vi "Controller Top Level.vi"(8 "error in (no error)":errorcluster) -> (0 "error out":errorcluster)   [LabVIEW 2020, in "Controller.lvlib"]
uses:
  Controller.lvlib
  Private Controls/Module Action.ctl
  Public Controls/Module Data Cluster.ctl
  Public Controls/Config.ctl
  c2d6bbf9-d574-4896-9299-2729cd30e33b.vi
  27c827a8-6ce2-46ff-b742-8397f53ceddc.vi
  e3555320-3669-4681-98ae-afe808cba037.vi
  16cb41ff-8f3c-4f22-bc48-50ffacbfc1d7.vi
  <vilib>/Utility/error.llb/Clear Errors.vi
  UI/UI.lvlib
  Error Handler/Error Handler.lvlib
panel:
  out "Action":T1
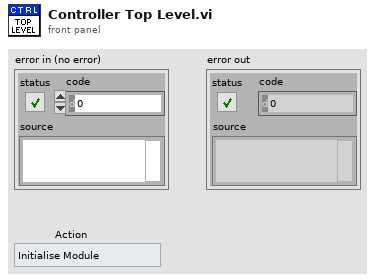
[diagram p1: front panel]
types:
  T1 = typedef "Controller.lvlib/Module Action.ctl" = enum16{"Initialise Module", "Connect", "Setup", "Pause", "Start", "Search Network", "Get Local", "Stop", "Wait: Time Elapsed", "Error", "Exit"}
  T2 = typedef "Controller.lvlib/Module Data Cluster.ctl" = cluster{"Pause?":bool, "Iteration":i32, "Time Elapsed?":bool, "Config":T3, "Local IP":string}
  T3 = typedef "Controller.lvlib/Config.ctl" = cluster{"Value":dbl}
  T4 = typedef "UI.lvlib/IP Address Response Type Def.ctl" = cluster{"Address":string, "Response":string, "Boolean":bool}
  T5 = typedef "UI.lvlib/IP Stats.ctl" = cluster{"Address":string, "Average Response Time":i32, "Loss %":i32, "Min Response Time":i32, "Max Response Time":i32, "Boolean":bool}
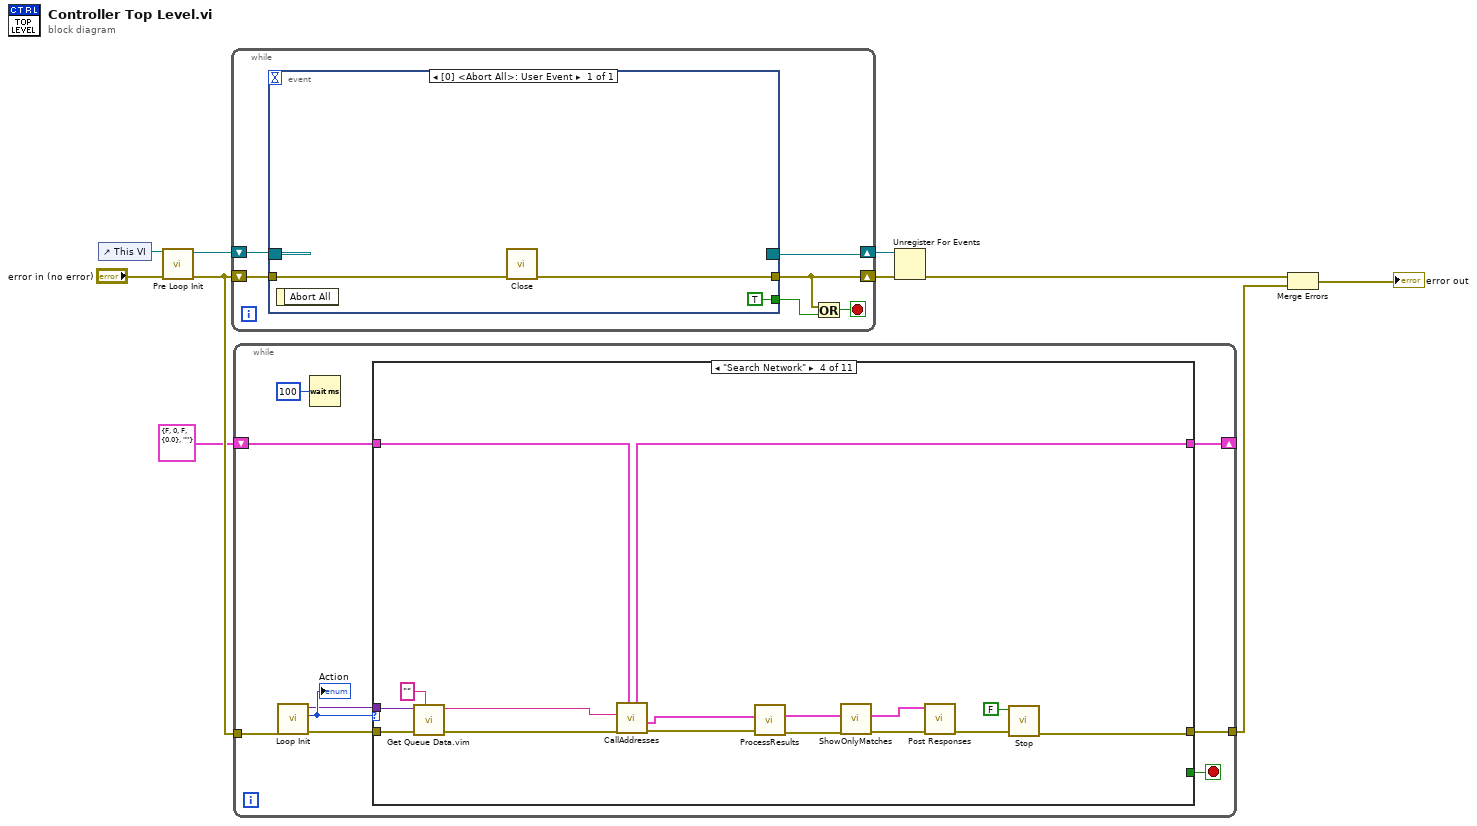
[diagram p0: block diagram]
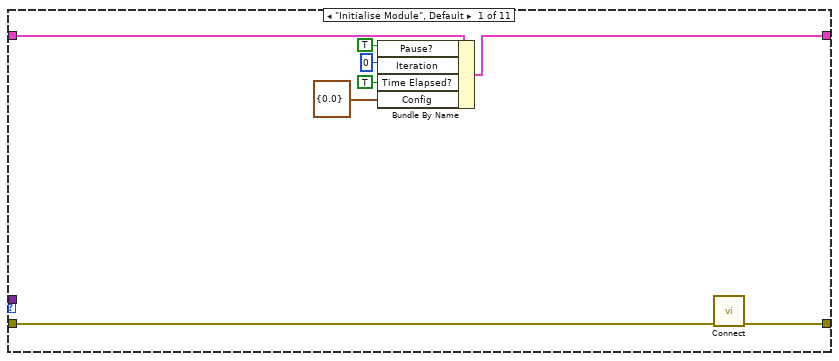
[diagram p2: hidden frame]
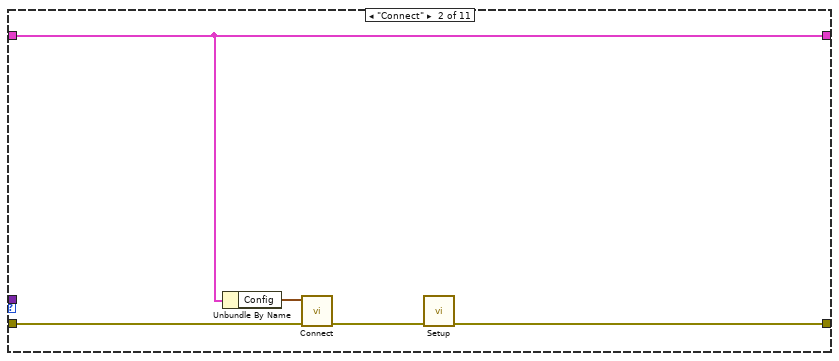
[diagram p3: hidden frame]
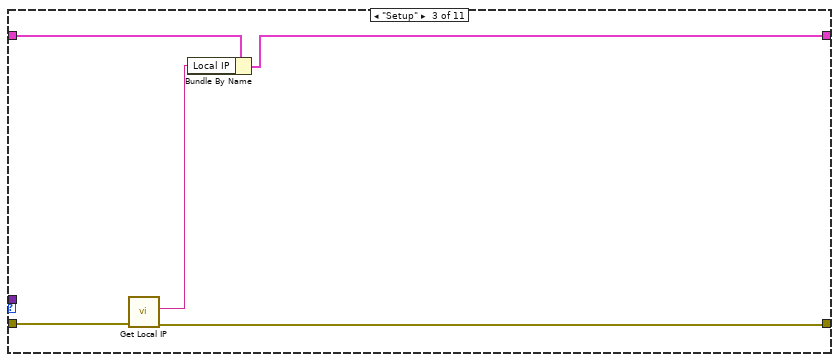
[diagram p4: hidden frame]
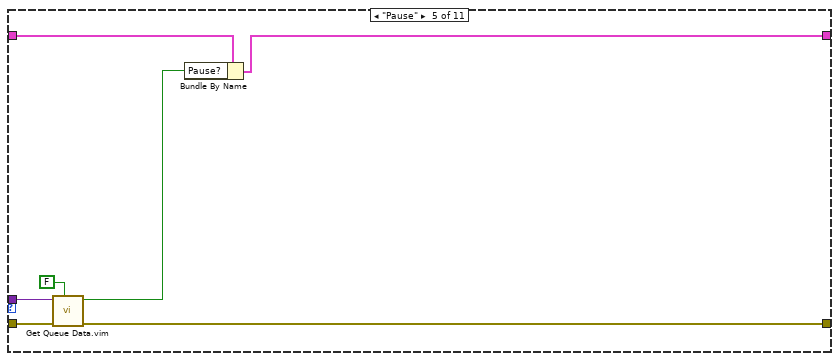
[diagram p5: hidden frame]
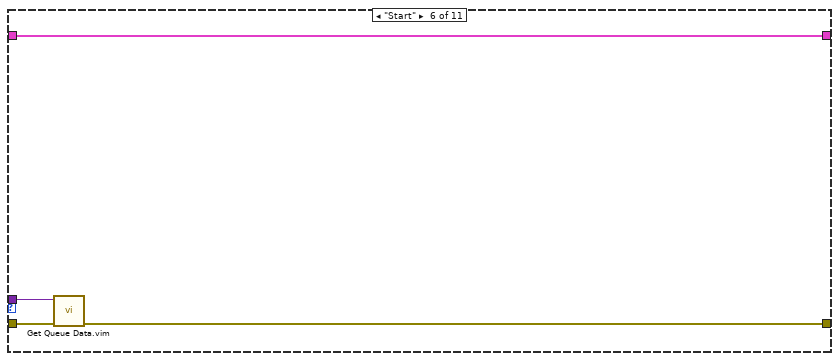
[diagram p6: hidden frame]
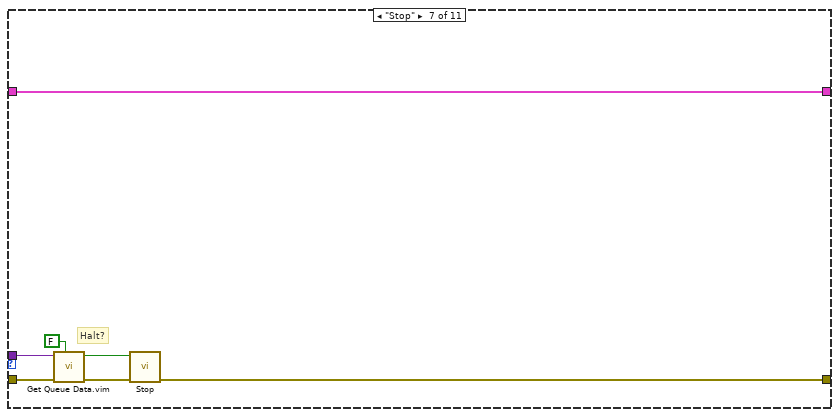
[diagram p7: hidden frame]
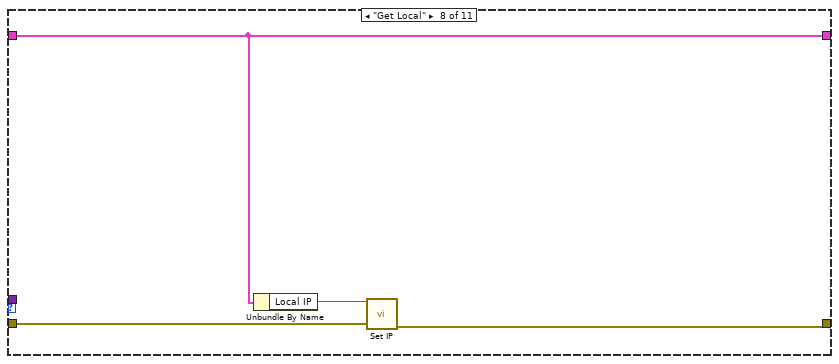
[diagram p8: hidden frame]
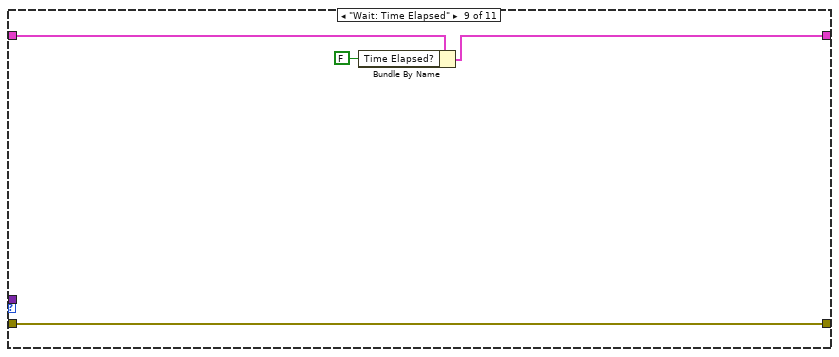
[diagram p9: hidden frame]
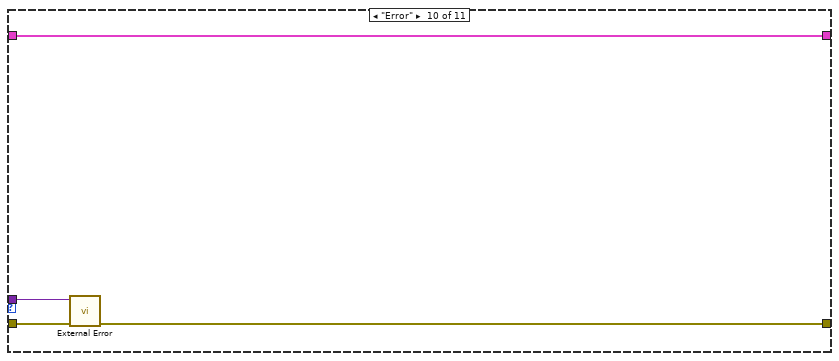
[diagram p10: hidden frame]
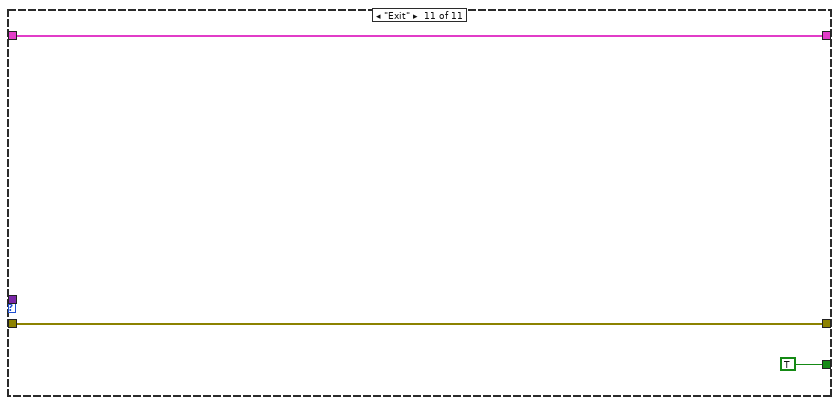
[diagram p11: hidden frame]
diagram:
  n1 = control-ref of="This VI"() -> (w4:refnum<vi>)
  n2 = call "Pre Loop Init.vi"("error in (no error)"="error in (no error)", "Ref In"=w4) -> ("error out"=w7:errorcluster, "Event Registration Refnum"=w6:refnum<event-registration>)  [unwired: 8 in]
  n3 = while {
    shift-right: [w13] -> w10
    shift-left: w7 -> [w12]
    shift-right: [w15] -> w5
    shift-left: w6 -> [w16]
    stop <- w14 stop-if-true
    n4 = event shown="[0] <Abort All>: User Event" {
      selector: w16 -> [_]
      dyn-events: [_] -> w15
      timeout: _ -> [_]
      tunnel: [w18] -> w13
      tunnel: w12 -> [w19]
      tunnel: [TRUE] -> w11
      event User Event {
        n5 = event-data() -> ()  [unwired: 1 in, 1 out]
        n6 = call "Close.vi"("error in (no error)"=w19) -> ("error out"=w18:errorcluster)  [unwired: 10 in]
      }
    }
    n7 = Or(x=w13, y=w11) -> (x .or. y?=w14:bool)
  }
  n8 = while {
    shift-right: [w23] -> _
    shift-left: T2 {"Pause?"=FALSE, "Iteration"=0, "Time Elapsed?"=FALSE, "Config"={"Value"=0.0}, "Local IP"=""} ("Module Data Cluster") -> [w24]
    tunnel: w7 -> [w27]
    tunnel: [w20] -> w8
    stop <- w22 stop-if-true
    n9 = call "Loop Init.vi"("error in (no error)"=w27) -> ("error out"=w25:errorcluster, "Action"=w26:T1, "Data"=w21:variant)  [unwired: 8 in]
    "Action" <- w26
    n10 = Wait (ms)(milliseconds to wait=u32 100) -> ()  [unwired: 1 out]
    n11 = case shown="\"Search Network\"" w26 {
      tunnel: w25 -> [w31 w40 w42 w59 w69 w72 w79 w83 w85 w91 w93]
      tunnel: w24 -> [w36 w41 w44 w62 w65 w73 w80 w84 w88 w92 w95]
      tunnel: [w35 w41 w45 w61 w64 w73 w80 w84 w87 w92 w95] -> w23
      tunnel: [_ _ _ _ _ _ _ _ _ _ TRUE] -> w22
      tunnel: w21 -> [_ _ _ w57 w68 w71 w78 _ _ w90 _]
      tunnel: [w29 w37 w46 w53 w63 w70 w76 w81 w85 w89 w93] -> w20
      frame "Initialise Module", Default {
        n12 = Bundle By Name(cluster=w36, "Pause?"=TRUE, "Iteration"=0, "Time Elapsed?"=TRUE, "Config"=T3 {"Value"=0.0}) -> (w35:T2)
        n13 = call "Connect.vi"("error in (no error)"=w31) -> ("error out"=w29:errorcluster)  [unwired: 10 in]
      }
      frame "Connect" {
        n14 = Unbundle By Name(w41) -> ("Config"=w39:T3)
        n15 = call "Connect.vi"("error in (no error)"=w40, "Data"=w39) -> ("error out"=w38:errorcluster)  [unwired: 9 in]
        n16 = call "Setup.vi"("error in (no error)"=w38) -> ("error out"=w37:errorcluster)  [unwired: 10 in]
      }
      frame "Setup" {
        n17 = call "Get Local IP.vi"("error in (no error)"=w42) -> ("error out"=w46:errorcluster, "Local IP"=w43:string)  [unwired: 9 in]
        n18 = Bundle By Name(cluster=w44, "Local IP"=w43) -> (w45:T2)
      }
      frame "Search Network" {
        n19 = call "Get Queue Data.vim"("Default Value"="", "error in"=w59, "Variant"=w57) -> ("error out"=w58:errorcluster, "Module Data"=w56:string)  [unwired: 7 in]
        n20 = call "CallAddresses.vi"("Module Cluster In"=w62, "error in (no error)"=w58, "Local Ip"=w56) -> ("error out"=w49:errorcluster, "Response Array"=w60:T4[], "Module Cluster Out"=w61:T2)  [unwired: 6 in]
        n21 = call "ProcessResults.vi"("error in (no error)"=w49, "Response Array"=w60) -> ("error out"=w48:errorcluster, "IP Stats"=w47:T5[])  [unwired: 8 in]
        n22 = call "ShowOnlyMatches.vi"("error in (no error)"=w48, "IP Stats In"=w47) -> ("error out"=w50:errorcluster, "IP Stats Out"=w52:T5[])  [unwired: 8 in]
        n23 = call "Post Responses.vi"("error in (no error)"=w50, "Data"=w52) -> ("error out"=w54:errorcluster)  [unwired: 9 in]
        n24 = call "Stop.vi"("error in (no error)"=w54, "Data"=FALSE) -> ("error out"=w53:errorcluster)  [unwired: 9 in]
      }
      frame "Pause" {
        n25 = call "Get Queue Data.vim"("Default Value"=FALSE, "error in"=w69, "Variant"=w68) -> ("error out"=w63:errorcluster, "Module Data"=w66:bool)  [unwired: 7 in]
        n26 = Bundle By Name(cluster=w65, "Pause?"=w66) -> (w64:T2)
      }
      frame "Start" {
        n27 = call "Get Queue Data.vim"("error in"=w72, "Variant"=w71) -> ("error out"=w70:errorcluster)  [unwired: 8 in, 1 out]
      }
      frame "Stop" {
        # "Halt?"
        n28 = call "Get Queue Data.vim"("Default Value"=FALSE, "error in"=w79, "Variant"=w78) -> ("error out"=w77:errorcluster, "Module Data"=w74:bool)  [unwired: 7 in]
        n29 = call "Stop.vi"("error in (no error)"=w77, "Data"=w74) -> ("error out"=w76:errorcluster)  [unwired: 9 in]
      }
      frame "Get Local" {
        n30 = Unbundle By Name(w84) -> ("Local IP"=w82:string)
        n31 = call "Set IP.vi"("error in (no error)"=w83, "Data"=w82) -> ("error out"=w81:errorcluster)  [unwired: 9 in]
      }
      frame "Wait: Time Elapsed" {
        n32 = Bundle By Name(cluster=w88, "Time Elapsed?"=FALSE) -> (w87:T2)
      }
      frame "Error" {
        n33 = call "External Error.vi"("error in (no error)"=w91, "Data"=w90) -> ("error out"=w89:errorcluster)  [unwired: 9 in]
      }
      frame "Exit" {
      }
    }
  }
  n34 = Unregister For Events(event registration refnum=w5, error in=w10) -> (error out=w9:errorcluster)
  n35 = Merge Errors(w9, w8) -> (→"error out":errorcluster)
